vi "OCV 4309 Finite.vi"(8 "error in":errorcluster, 10 "Rate (Hz)":dbl=1000.0 format="%#_13g") -> (0 "error out":errorcluster, 1 "Clear Time (ms)":u32=1599, 2 "Voltage":sgl[](array[numeric]) format="%#_8g")   [LabVIEW 2019]
doc: "This example demonstrates how to enable the Chop feature in a continuously acquire buffered voltage measurement using a DAQmx device.\n\nFor instructions on how to connect your signals to the DAQ device, refer to your device documentation."
panel:
  in  "# of Triggers":i32=10
  out "# of Triggers Sent":i32
  out "Read Time (ms)":u32[](array[numeric])
  out "Trigger Time (ms)":u32[](array[numeric])
  out "Voltage":sgl[][](array[numeric]) format="%#_8g"
  out "Config Time":u32
  out "Position vs Trigger":cluster{dbl[], dbl[]}[](graph)
  out "Read Time (ms)":u32=46
  out "Trigger Time (ms)":u32=46
  in  "Chop":bool=TRUE
  in  "Max Voltage":dbl=10.0
  in  "Min Voltage":dbl=-10.0
  in  "Physical Channel":tag="4309/ai0:4"
  # "DAQmx Settings"
  # "On (T)"
  # "Off (F)"
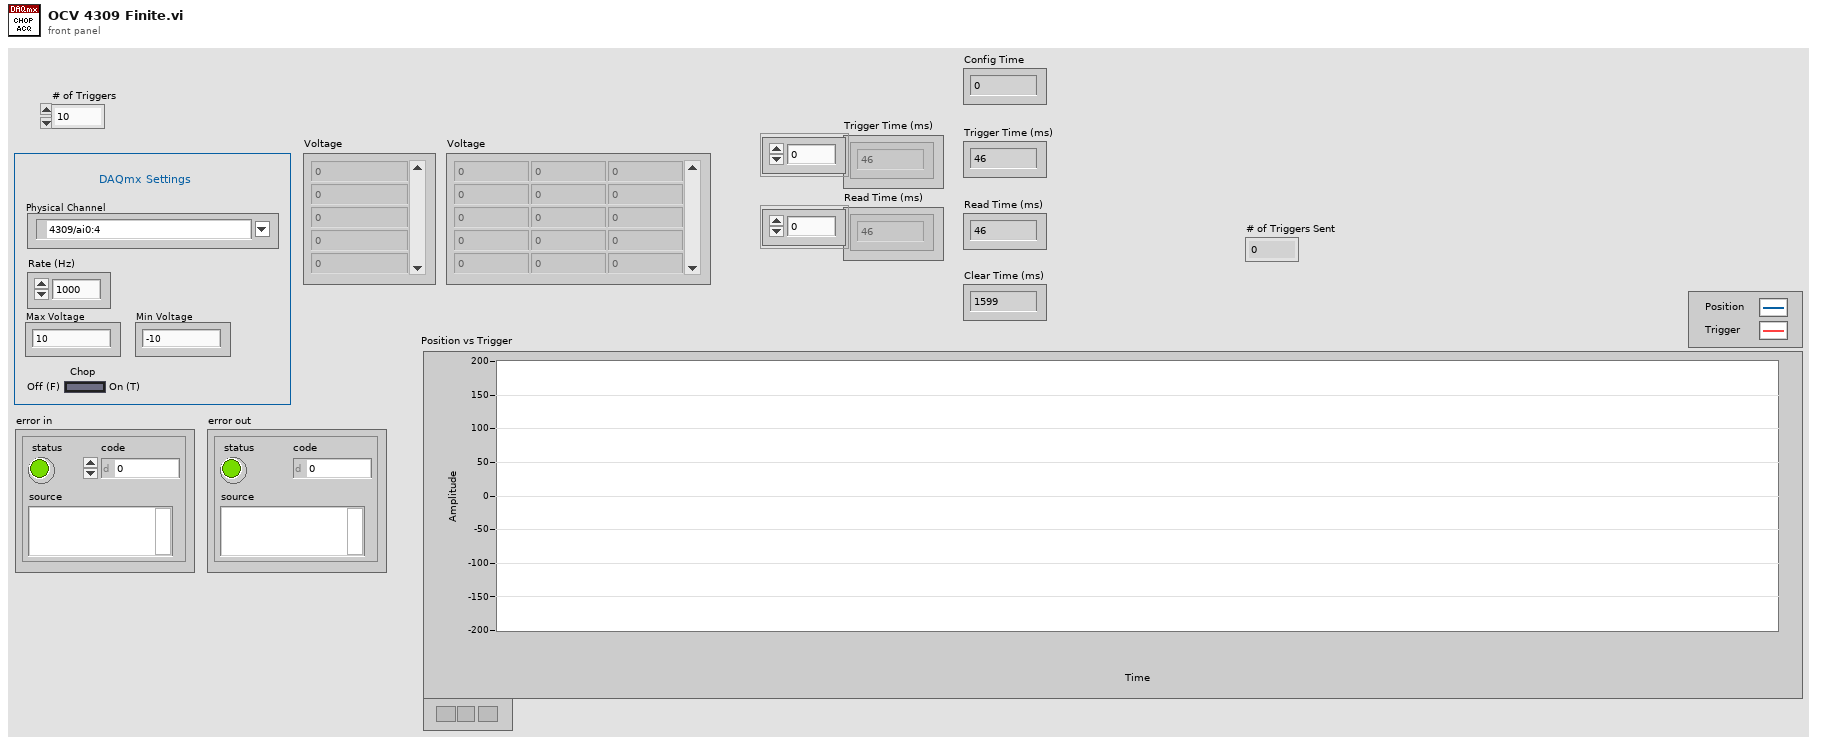
[diagram p1: front panel]
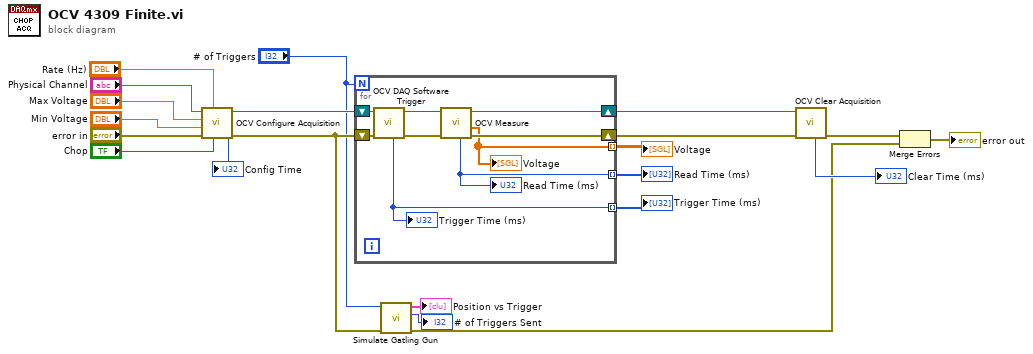
[diagram p0: block diagram]
diagram:
  n1 = call "OCV Configure Acquisition.vi"("Chop"="Chop", "Rate (Hz)"="Rate (Hz)", "error in (no error)"="error in", "Min Voltage"="Min Voltage", "Max Voltage"="Max Voltage", "Physical Channel"="Physical Channel") -> ("error out"=w4:errorcluster, "Refnum out"=w14:refnum<k21>, "Config Time"=→"Config Time":u32)  [unwired: 3 in]
  n2 = for {
    N: "# of Triggers" -> [_]
    shift-right: [w29] -> w15
    shift-left: w14 -> [w28]
    shift-right: [w30] -> w21
    shift-left: w4 -> [w26]
    tunnel: [w24] -> w7 mode=indexing
    tunnel: [w23] -> w6 mode=indexing
    tunnel: [w22] -> w5 mode=indexing
    n3 = call "OCV DAQ Software Trigger.vi"("error in (no error)"=w26, "Refnum in"=w28) -> ("error out"=w25:errorcluster, "Refnum out"=w27:refnum<k21>, "Trigger Time (ms)"=w22:u32)  [unwired: 7 in]
    "Trigger Time (ms)" <- w22
    n4 = call "OCV Measure.vi"("error in (no error)"=w25, "Refnum in"=w27) -> ("error out"=w30:errorcluster, "Voltage"=w24:sgl[], "Refnum out"=w29:refnum<k21>, "Read Time (ms)"=w23:u32)  [unwired: 6 in]
    "Voltage" <- w24
    "Read Time (ms)" <- w23
  }
  "Voltage" <- w7
  "Trigger Time (ms)" <- w5
  "Read Time (ms)" <- w6
  n5 = call "Simulate Gatling Gun.vi"("error in (no error)"=w4, "# of Triggers"="# of Triggers") -> ("error out"=w8:errorcluster, "# of Triggers Sent"=→"# of Triggers Sent":i32, "Position vs Trigger"=→"Position vs Trigger":cluster{dbl[], dbl[]}[])  [unwired: 7 in]
  n6 = call "OCV Clear Acquisition.vi"("error in (no error)"=w21, "Refnum in"=w15) -> ("error out"=w10:errorcluster, "Clear Time (ms)"=→"Clear Time (ms)":u32)  [unwired: 8 in]
  n7 = Merge Errors(w10, w8) -> (→"error out":errorcluster)
